vi "Parse Response JSON.vi"(8 "error in (no error)":errorcluster, 10 "Response JSON":string, 11 "RGetStreamStatus in":refnum<class "RGetStreamStatus.lvclass">) -> (0 "error out":errorcluster, 3 "RGetStreamStatus out":refnum<class "RGetStreamStatus.lvclass">)   [LabVIEW 2022 SP3, in "obs-websocket-lv.lvlib" / "RGetStreamStatus.lvclass"]
uses:
  RGetStreamStatus.lvclass
  RGetStreamStatus.lvclass/RGetStreamStatus.ctl
  <vilib>/IlluminatedG/lv-web-crypto/lv-json/JSON/JSON.lvlib
  Stream Status.ctl
  obs-websocket-lv.lvlib
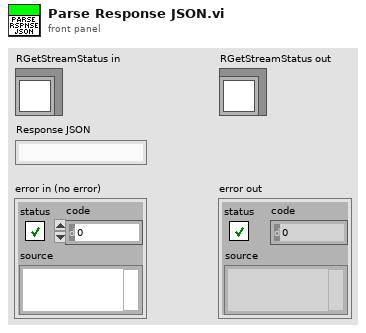
[diagram p1: front panel]
types:
  T1 = typedef "obs-websocket-lv.lvlib/Stream Status.ctl" = cluster{"Active":bool, "Reconnecting":bool, "Timecode":string, "Duration mS":u32, "Bytes":u32, "Skipped Frames":u32, "Total Frames":u32}
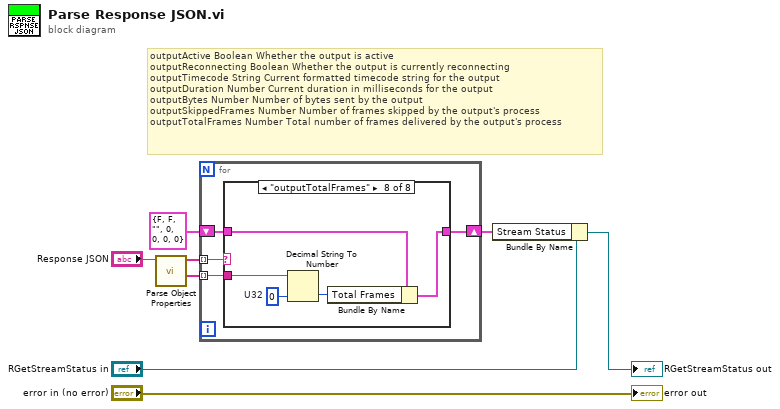
[diagram p0: block diagram]
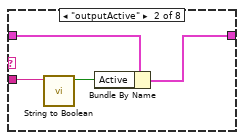
[diagram p3: hidden frame]
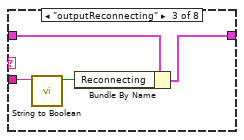
[diagram p4: hidden frame]
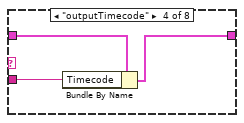
[diagram p5: hidden frame]
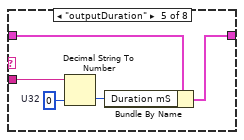
[diagram p6: hidden frame]
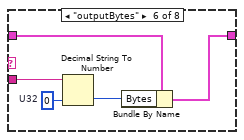
[diagram p7: hidden frame]
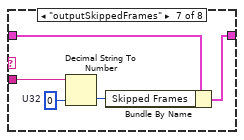
[diagram p8: hidden frame]
diagram:
  # "outputActive\tBoolean\tWhether the output is active\noutputReconnecting\tBoolean\tWhether the output is currently reconnecting\noutputTimecode\tString\tCurrent formatted timecode string for the output\noutputDuration\tNumber\tCurrent duration in milliseconds for the output\noutputBytes\tNumber\tNumber of bytes sent by the output\noutputSkippedFrames\tNumber\tNumber of frames skipped by the output's process\noutputTotalFrames\tNumber\tTotal number of frames delivered by the output's process"
  n1 = call <vilib>:"Parse Object Properties.vi"("JSON String"="Response JSON") -> ("Values"=w5:string[], "Keys"=w4:string[])  [unwired: 7 in, 2 out]
  n2 = for {
    tunnel: w5 -> [w11] mode=indexing
    tunnel: w4 -> [w12] mode=indexing
    shift-right: [w9] -> w1
    shift-left: T1 {"Active"=FALSE, "Reconnecting"=FALSE, "Timecode"="", "Duration mS"=0, "Bytes"=0, "Skipped Frames"=0, "Total Frames"=0} ("Stream Status") -> [w10]
    n3 = case shown="\"outputTotalFrames\"" w12 {
      tunnel: w11 -> [_ w17 w19 w23 w28 w32 w35 w40]
      tunnel: w10 -> [w13 w16 w21 w24 w29 w31 w36 w41]
      tunnel: [w13 w14 w20 w22 w25 w30 w37 w42] -> w9
      frame Default {
      }
      frame "outputActive" {
        n4 = call <vilib>:"String to Boolean.vi"("Bool String"=w17) -> ("Boolean"=w15:bool)  [unwired: 10 in]
        n5 = Bundle By Name(cluster=w16, "Active"=w15) -> (w14:T1)
      }
      frame "outputReconnecting" {
        n6 = call <vilib>:"String to Boolean.vi"("Bool String"=w19) -> ("Boolean"=w18:bool)  [unwired: 10 in]
        n7 = Bundle By Name(cluster=w21, "Reconnecting"=w18) -> (w20:T1)
      }
      frame "outputTimecode" {
        n8 = Bundle By Name(cluster=w24, "Timecode"=w23) -> (w22:T1)
      }
      frame "outputDuration" {
        w26 = u32 0  # U32
        n9 = Decimal String To Number(string=w28, default (0L)=w26) -> (number=w27:u32)  [unwired: 1 in, 1 out]
        n10 = Bundle By Name(cluster=w29, "Duration mS"=w27) -> (w25:T1)
      }
      frame "outputBytes" {
        w33 = u32 0  # U32
        n11 = Decimal String To Number(string=w32, default (0L)=w33) -> (number=w34:u32)  [unwired: 1 in, 1 out]
        n12 = Bundle By Name(cluster=w31, "Bytes"=w34) -> (w30:T1)
      }
      frame "outputSkippedFrames" {
        w38 = u32 0  # U32
        n13 = Decimal String To Number(string=w35, default (0L)=w38) -> (number=w39:u32)  [unwired: 1 in, 1 out]
        n14 = Bundle By Name(cluster=w36, "Skipped Frames"=w39) -> (w37:T1)
      }
      frame "outputTotalFrames" {
        w43 = u32 0  # U32
        n15 = Decimal String To Number(string=w40, default (0L)=w43) -> (number=w44:u32)  [unwired: 1 in, 1 out]
        n16 = Bundle By Name(cluster=w41, "Total Frames"=w44) -> (w42:T1)
      }
    }
  }
  n17 = Bundle By Name(cluster="RGetStreamStatus in", "Stream Status"=w1) -> (→"RGetStreamStatus out":refnum<class "RGetStreamStatus.lvclass">)
  "error out" <- "error in (no error)"
